vi "在线监测仪器仪表参数.vi"() -> ()   [LabVIEW 2016]
panel:
  in  "浊度参数":T1
  in  "电导率参数":T1
  in  "溶解氧参数":T1
  in  "PH参数":T1
  in  "水温参数":T1
  in  "CODCr参数":T1
  in  "总氮参数":T1
  in  "总磷参数":T1
  in  "氨氮参数":T1
  in  "CODMn参数":T1
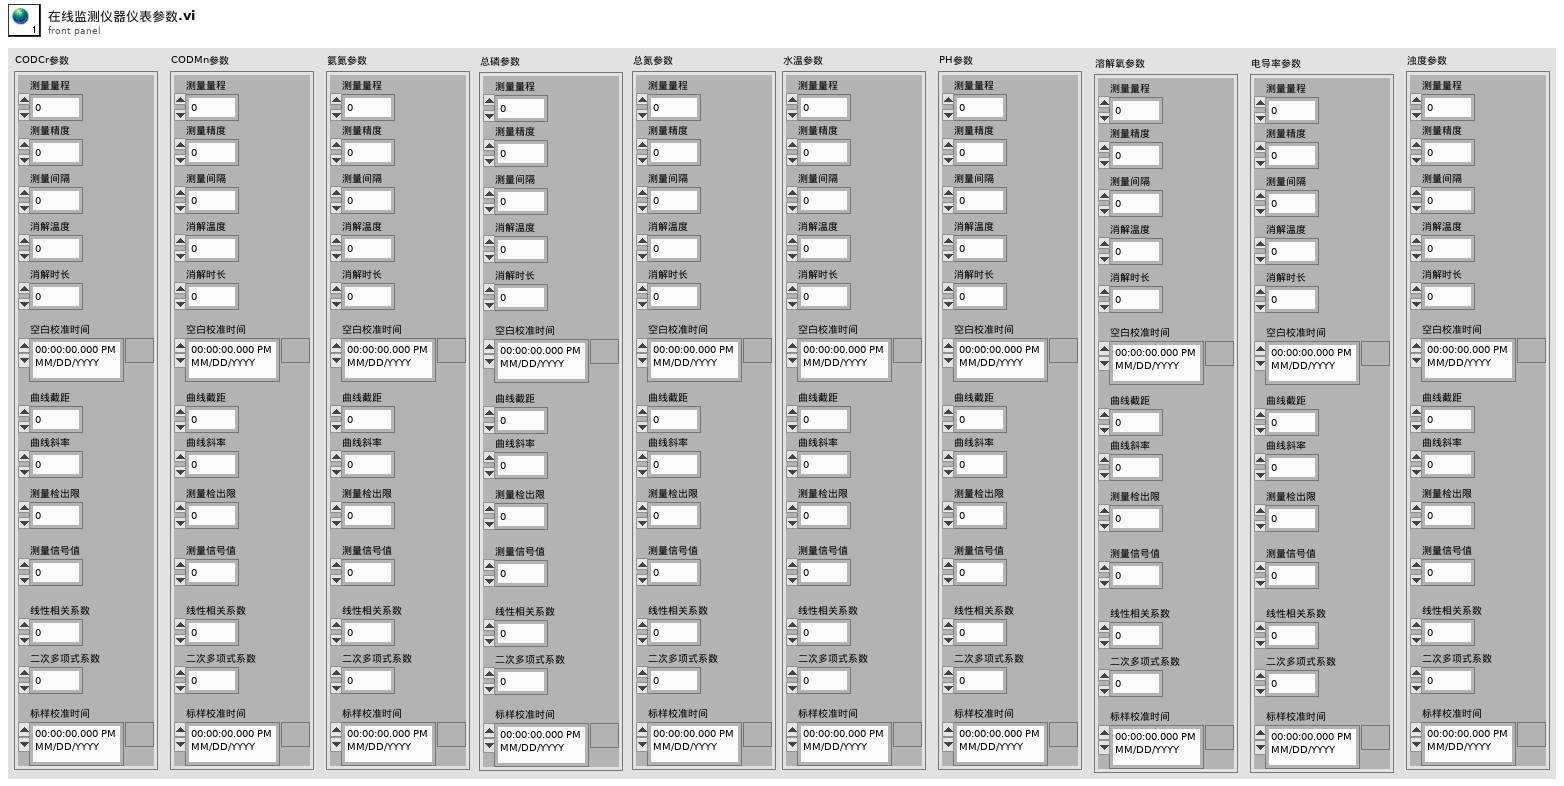
[diagram p1: front panel]
types:
  T1 = cluster{"测量量程":dbl, "测量精度":dbl, "测量间隔":dbl, "消解温度":dbl, "消解时长":dbl, "空白校准时间":timestamp, "曲线截距":dbl, "曲线斜率":dbl, "测量检出限":dbl, "测量信号值":dbl, "线性相关系数":dbl, "二次多项式系数":dbl, "标样校准时间":timestamp}
diagram:
